vi "Array to Multi Ch Waveforms.vi"(8 "channel names":string[](array[string]), 10 "dt":dbl, 11 "array":dbl[](array[numeric])) -> (3 "waveforms":waveform(dbl)[](array[waveform]))   [LabVIEW 2021]
uses:
  51ac07c7-d09d-49cc-87c4-ca496b6be0c5.vi
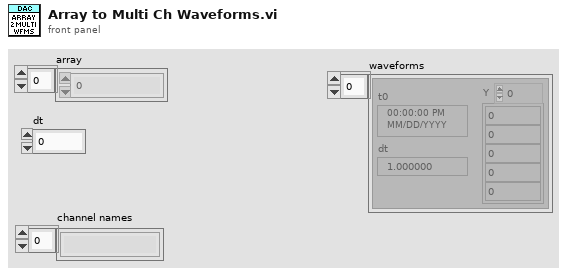
[diagram p1: front panel]
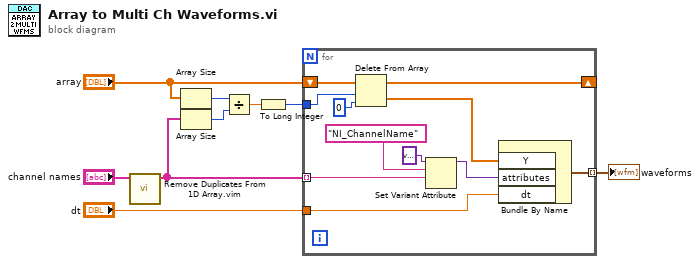
[diagram p0: block diagram]
diagram:
  n1 = call "Remove Duplicates From 1D Array.vim"("array"="channel names") -> ("array with duplicates removed"=w1:string[])  [unwired: 10 in]
  n2 = Array Size(array="array") -> (size(s)=w9:i32)
  n3 = Array Size(array=w1) -> (size(s)=w8:i32)
  n4 = Divide(x=w9, y=w8) -> (x/y=w6:dbl)
  n5 = To Long Integer(number=w6) -> (32bit integer=w5:i32)
  n6 = for {
    shift-right: [w19] -> _
    shift-left: "array" -> [w20]
    tunnel: w5 -> [w17]
    tunnel: w1 -> [w15] mode=indexing
    tunnel: "dt" -> [w10]
    tunnel: [w13] -> w3 mode=indexing
    n7 = Delete From Array(array=w20, length=w17, index=0) -> (deleted portion=w11:dbl[], array with subset deleted=w19:dbl[])
    n8 = Set Variant Attribute(Variant=variant ("variant"), name="NI_ChannelName", value=w15) -> (Variant out=w16:variant)  [unwired: 1 in, 2 out]
    n9 = Bundle By Name("Y"=w11, "attributes"=w16, "dt"=w10) -> (w13:waveform(dbl))  [unwired: 1 in]
  }
  "waveforms" <- w3
